vi "Evaluate Part 1.vi"() -> ()   [LabVIEW 2021]
panel:
  out "Numeric":u64
  in  "Input":string="rn=1,cm-,qp=3,cm=2,qp-,pc=4,ot=9,ab=5,pc-,pc=6,ot=7"
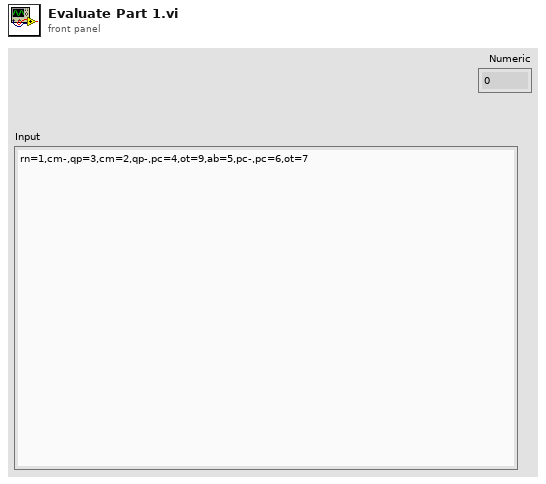
[diagram p1: front panel]
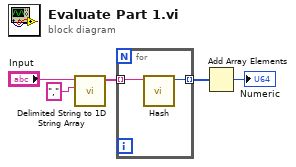
[diagram p0: block diagram]
diagram:
  n1 = call <vilib>:"Delimited String to 1D String Array.vi"("delimiter"=",", "delimited string"="Input") -> ("string array"=w2:string[])  [unwired: 9 in]
  n2 = for {
    tunnel: [w6] -> w5 mode=indexing
    tunnel: w2 -> [w7] mode=indexing
    n3 = call "Hash.vi"("String"=w7) -> ("Numeric"=w6:u64)  [unwired: 10 in]
  }
  n4 = Add Array Elements(numeric array=w5) -> (sum=→"Numeric":u64)
